vi "SRV_SensorsQueue_Enqueue Element.vi"(6 "Ignore Error 1? (F)":bool, 8 "error in (no error)":errorcluster, 9 "Data":variant, 10 "Command":string) -> (0 "error out":errorcluster)   [LabVIEW 2014]
uses:
  Support/SRV_Command-Data Queue Data Type.ctl
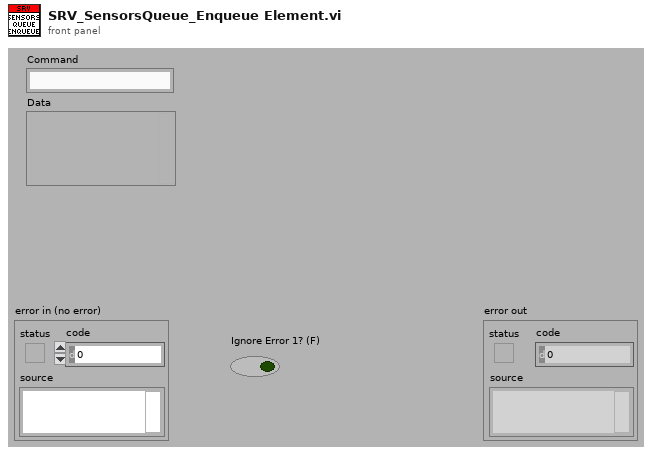
[diagram p1: front panel]
types:
  T1 = typedef "SRV_Command-Data Queue Data Type.ctl" = cluster{"Command":string, "Data":variant}
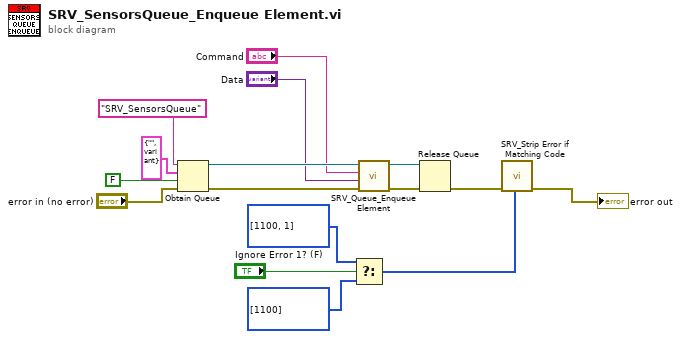
[diagram p0: block diagram]
diagram:
  n1 = Obtain Queue(name (unnamed)="SRV_SensorsQueue", element data type=T1 {"Command"="", "Data"=variant} ("Queue Data Type"), create if not found? (T)=FALSE, error in (no error)="error in (no error)") -> (queue out=w12:refnum<queue>, error out=w11:errorcluster)  [unwired: 1 in, 1 out]
  n2 = Select(t=i32[] [1100, 1] ("Strip Codes"), s="Ignore Error 1? (F)", f=i32[] [1100] ("Strip Codes")) -> (s? t:f=w2:i32[])
  n3 = call "SRV_Queue_Enqueue Element.vi"("error in (no error)"=w11, "Data"="Data", "Command"="Command", "Command-Data Queue"=w12) -> ("error out"=w9:errorcluster, "Command-Data Queue out"=w10:refnum<queue>)  [unwired: 5 in, 1 out]
  n4 = Release Queue(queue=w10, error in (no error)=w9) -> (error out=w6:errorcluster)  [unwired: 1 in, 2 out]
  n5 = call "SRV_Strip Error if Matching Code.vi"("error in (no error)"=w6, "Strip Codes"=w2) -> ("error out"=→"error out":errorcluster)  [unwired: 8 in]
